vi "New.vi"(6 "Creator Queue":refnum<data-value>, 8 "Creator Queue Alias":string, 9 "Self Queue":refnum<data-value>, 10 "Self Queue Alias":string) -> (0 "error out":errorcluster, 2 "Queue Mailbox":refnum<data-value>)   [LabVIEW 2021, in "jettl.lvlib" / "Queue Mailbox.lvlib"]
uses:
  Queue Mailbox.lvlib
  Queue Mailbox/Queue Mailbox.lvclass
  Msg Strategy/Msg Strategy.lvclass
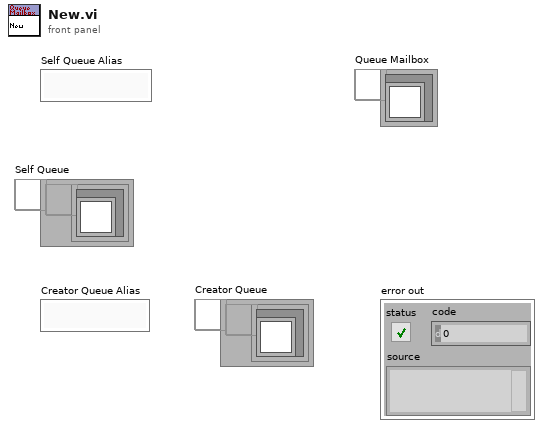
[diagram p1: front panel]
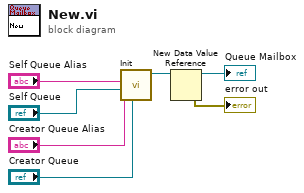
[diagram p0: block diagram]
diagram:
  n1 = call "Init.vi"("Creator Queue"="Creator Queue", "Creator Queue Alias"="Creator Queue Alias", "Self Queue"="Self Queue", "Self Queue Alias"="Self Queue Alias") -> ("Queue Mailbox out"=w5:refnum<class "Queue Mailbox.lvclass">)  [unwired: 7 in]
  n2 = New Data Value Reference(data value=w5) -> (data value reference=→"Queue Mailbox":refnum<data-value>, error out=→"error out":errorcluster)  [unwired: 1 in]
